vi "Read Temperatures.vi"(8 "error in":errorcluster, 11 "Thermometer Multichannel Worker in":refnum<class "Thermometer Multichannel Worker.lvclass">) -> (0 "error out":errorcluster, 3 "Thermometer Multichannel Worker out":refnum<class "Thermometer Multichannel Worker.lvclass">)   [LabVIEW 2024, in "Thermometer Multichannel Worker.lvlib" / "Thermometer Multichannel Worker.lvclass"]
uses:
  Thermometer Multichannel Worker.lvclass
  Thermometer Multichannel Worker.lvclass/Thermometer Multichannel Worker.ctl
  Interfaces/IRead Temperature Multichannel/IRead Temperature Multichannel.lvclass
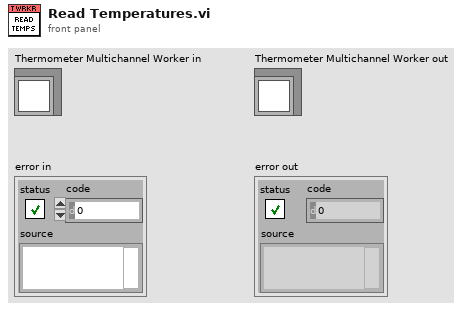
[diagram p1: front panel]
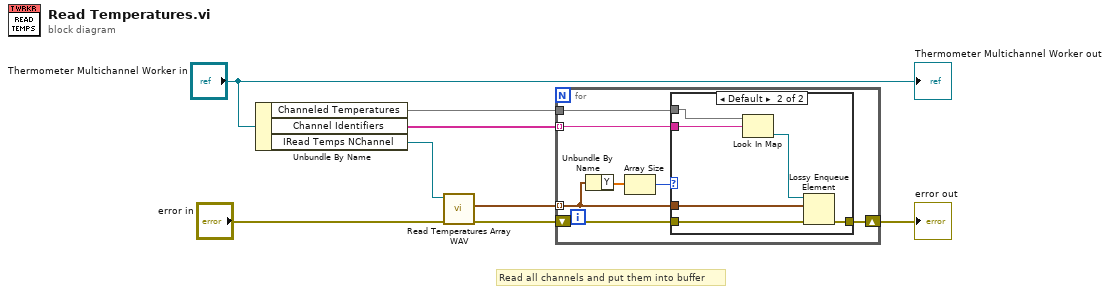
[diagram p0: block diagram]
diagram:
  # "Read all channels and put them into buffer"
  n1 = Unbundle By Name("Thermometer Multichannel Worker in") -> ("Channeled Temperatures"=w2:map{string, refnum<queue>}, "Channel Identifiers"=w1:string[], "IRead Temps NChannel"=w4:refnum<class "IRead Temperature Multichannel.lvclass">)
  n2 = call-dynamic "Read Temperatures Array WAV.vi"("error in"="error in", "IRead Temperature Multichannel in"=w4) -> ("error out"=w5:errorcluster, "Temperatures"=w3:waveform(dbl)[])  [unwired: 7 in, 1 out]
  n3 = for {
    shift-right: [w14] -> w7
    shift-left: w5 -> [w15]
    tunnel: w3 -> [w11] mode=indexing
    tunnel: w2 -> [w13]
    tunnel: w1 -> [w12] mode=indexing
    n4 = Unbundle By Name(w11) -> ("Y"=w9:dbl[])
    n5 = Array Size(array=w9) -> (size(s)=w10:i32)
    n6 = case shown="Default" w10 {
      tunnel: w15 -> [w16 w22]
      tunnel: [w16 w21] -> w14
      tunnel: w13 -> [_ w20]
      tunnel: w12 -> [_ w19]
      tunnel: w11 -> [_ w17]
      frame 0 {
      }
      frame Default {
        n7 = Look In Map(map=w20, key=w19) -> (value=w18:refnum<queue>)  [unwired: 1 in, 1 out]
        n8 = Lossy Enqueue Element(queue=w18, element=w17, error in (no error)=w22) -> (error out=w21:errorcluster)  [unwired: 3 out]
      }
    }
  }
  "error out" <- w7
  "Thermometer Multichannel Worker out" <- "Thermometer Multichannel Worker in"
